vi "series_parser_tester.vi"() -> ()   [LabVIEW 2024]
uses:
  definitions/seriesInfo.ctl
  series_class/series_class.lvclass
  series_class/series_class.lvclass/series_class.ctl
  comic_class/comic_class.lvclass
panel:
  out "error out":errorcluster
  in  "url":string
  out "paginated count":i32
  out "seriesInfo":T1
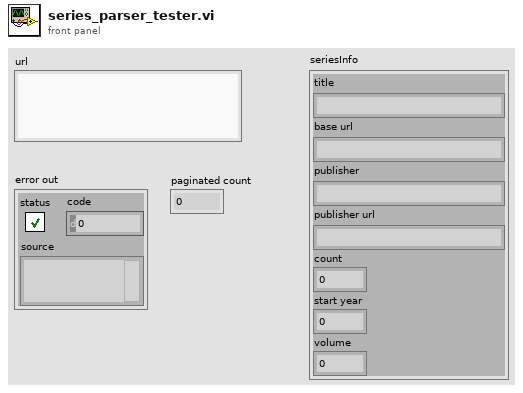
[diagram p1: front panel]
types:
  T1 = typedef "seriesInfo.ctl" = cluster{"title":string, "base url":string, "publisher":string, "publisher url":string, "count":i32, "start year":i32, "volume":i32}
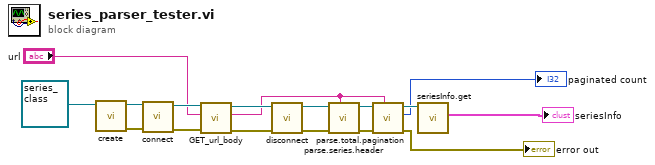
[diagram p0: block diagram]
diagram:
  n1 = call "create.vi"("comic_class in"=refnum<class "series_class.lvclass"> refnum ("ComicVine_class in")) -> ("error out"=w12:errorcluster, "comic_class out"=w13:refnum<class "series_class.lvclass">)  [unwired: 9 in]
  n2 = call-dynamic "connect.vi"("error in (no error)"=w12, "comic_class in"=w13) -> ("error out"=w11:errorcluster, "comic_class out"=w9:refnum<class "series_class.lvclass">)  [unwired: 8 in]
  n3 = call-dynamic "GET_url_body.vi"("error in (no error)"=w11, "url"="url", "comic_class in"=w9) -> ("error out"=w10:errorcluster, "body"=w7:string, "comic_class out"=w8:refnum<class "series_class.lvclass">)  [unwired: 6 in]
  n4 = call-dynamic "disconnect.vi"("error in (no error)"=w10, "comic_class in"=w8) -> ("error out"=w5:errorcluster, "comic_class out"=w1:refnum<class "series_class.lvclass">)  [unwired: 8 in]
  n5 = call "parse.series.header.vi"("series body"=w7, "error in (no error)"=w5, "ComicVine_class in"=w1) -> ("error out"=w4:errorcluster, "ComicVine_class out"=w16:refnum<class "series_class.lvclass">)  [unwired: 7 in]
  n6 = call "parse.total.pagination.vi"("series body"=w7, "error in (no error)"=w4, "ComicVine_class in"=w16) -> ("error out"=→"error out":errorcluster, "paginated count"=→"paginated count":i32, "ComicVine_class out"=w15:refnum<class "series_class.lvclass">)  [unwired: 6 in]
  n7 = call "seriesInfo.get.vi"("ComicVine_class in"=w15) -> ("seriesInfo"=→"seriesInfo":T1)  [unwired: 9 in, 1 out]
